vi "Destruct Messenger.vi"(8 "error in (no error)":errorcluster, 11 "Map Tree Queue Messenger Component in":refnum<class "Map Tree Queue Messenger.lvclass">) -> (0 "error out":errorcluster, 3 "Map Tree Queue Messenger Component out":refnum<class "Map Tree Queue Messenger.lvclass">)   [LabVIEW 2019, in "Map Tree Queue Messenger.lvclass"]
uses:
  Map Tree Queue Messenger.lvclass
  C:/Users/User/Desktop/Bussiness/Multi SPIM/General Library/Ancestor Class/Messenger/Messenger Map Composite/Messenger Map Composite.lvclass
  Map Tree Queue Messenger.lvclass/Map Tree Queue Messenger.ctl
  Ancestor Class/Messenger/Messenger Map Composite/Messenger Map Composite.lvclass/Messenger Map Composite.ctl
  Ancestor Class/Messenger/Messenger Map Composite/Public Data/Read Child Nodes.vi
  Ancestor Class/Messenger/Messenger/Messenger.lvclass
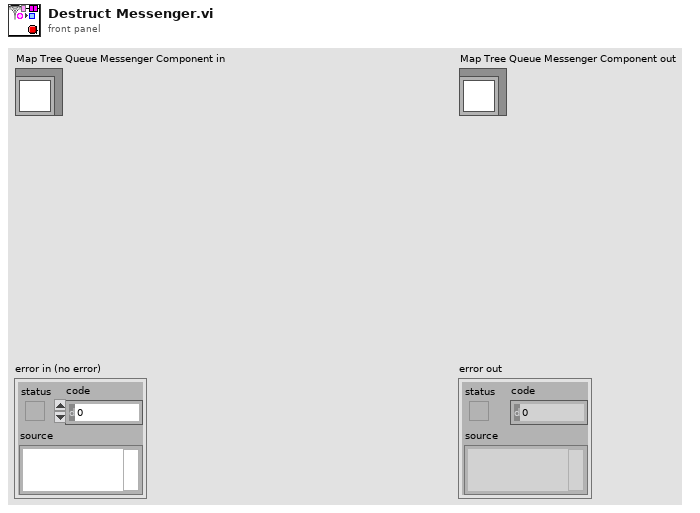
[diagram p1: front panel]
types:
  T1 = typedef "Message Queue.ctl" = refnum<queue>
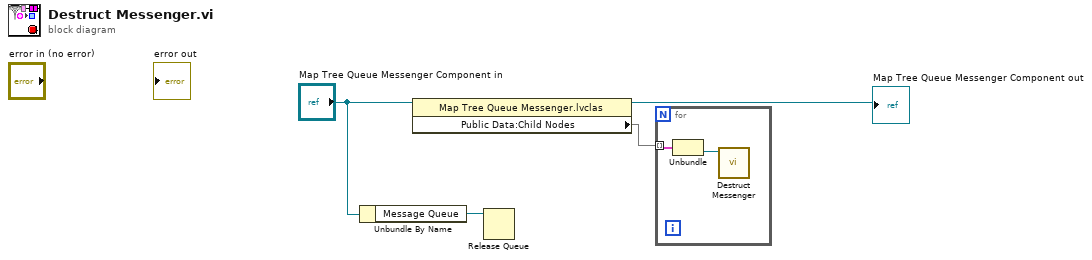
[diagram p0: block diagram]
diagram:
  n1 = Unbundle By Name("Map Tree Queue Messenger Component in") -> ("Message Queue"=w4:T1)
  n2 = property class="Map Tree Queue Messenger.lvclas"(reference="Map Tree Queue Messenger Component in") -> (reference out=→"Map Tree Queue Messenger Component out":refnum<class "Map Tree Queue Messenger.lvclass">, "Public Data:Child Nodes"=w3:map{i64, refnum<class "Messenger.lvclass">})  [unwired: 1 in, 1 out]
  n3 = Release Queue(queue=w4) -> ()  [unwired: 2 in, 3 out]
  n4 = for {
    tunnel: w3 -> [w6] mode=indexing
    n5 = Unbundle(w6) -> ("Messenger"=w5:refnum<class "Messenger.lvclass">)  [unwired: 1 out]
    n6 = call-dynamic "Destruct Messenger.vi"("Messenger Component in"=w5) -> ()  [unwired: 9 in, 2 out]
  }
